vi "Multiscale Wavelet.vi"() -> ()   [LabVIEW 2023]
uses:
  SubVIs/WaveLet Param Cluster Typedef.ctl
  SubVIs/WaveLet Ramp Param Cluster Typedef.ctl
  Images/_Images.ctl
  <vilib>/addons/_Advanced Signal Processing/NI_AdvSigProcWA.lvlib
  <vilib>/vision/NI_Vision_Development_Module.lvlib
panel:
  in  "Overall Contrast":dbl=0.7
  out "Histogram Original":T1(graph)
  out "Histogram Reconstructed":T1(graph)
  in  "Multiplier":dbl[](array[slide])=[220.55384826660156, 212.6769256591797, 192.984619140625, 252.06153869628906, 283.5692443847656, 319.015380859375, 252.06153869628906, 236.3076934814453, 181.1692352294922, 110.27692413330078, 129.96923076923076, 102.4000015258789] scale=0.0..512.0
  in  "Power":dbl[](array[slide])=[0.38461539149284363, 0.4307692348957062, 0.38461539149284363, 0.5230769515037537, 0.42307692766189575, 0.5538461804389954, 0.6461538672447205, 0.6153846383094788, 0.6153846383094788, 0.6000000238418579, 0.4000000059604645, 0.4000000059604645] scale=0.0..2.0
  in  "Image":T2=enum."Part1"
  in  "Amplitudes & Widths":T3[][](array[typedef])=[[{"Amplitude"=1.0, "Width"=1.0}, {"Amplitude"=0.1, "Width"=1.0}, {"Amplitude"=0.1, "Width"=1.0}], [{"Amplitude"=1.0, "Width"=1.0}, {"Amplitude"=1.0, "Width"=1.0}, {"Amplitude"=1.0, "Width"=1.0}], [{"Amplitude"=1.0, "Width"=1.0}, {"Amplitude"=1.0, "Width"=1.0}, {"Amplitude"=1.0, "Width"=1.0}], [{"Amplitude"=1.0, "Width"=1.0}, {"Amplitude"=1.0, "Width"=1.0}, {"Amplitude"=1.0, "Width"=1.0}], [{"Amplitude"=1.0, "Width"=1.0}, {"Amplitude"=1.0, "Width"=1.0}, {"Amplitude"=1.0, "Width"=1.0}], [{"Amplitude"=1.0, "Width"=1.0}, {"Amplitude"=1.0, "Width"=1.0}, {"Amplitude"=1.0, "Width"=1.0}], [{"Amplitude"=1.0, "Width"=1.0}, {"Amplitude"=1.0, "Width"=1.0}, {"Amplitude"=1.0, "Width"=1.0}], [{"Amplitude"=1.0, "Width"=1.0}, {"Amplitude"=1.0, "Width"=1.0}, {"Amplitude"=1.0, "Width"=1.0}], [{"Amplitude"=1.0, "Width"=1.0}, {"Amplitude"=1.0, "Width"=1.0}, {"Amplitude"=1.0, "Width"=1.0}], [{"Amplitude"=1.0, "Width"=1.0}, {"Amplitude"=1.0, "Width"=1.0}, {"Amplitude"=1.0, "Width"=1.0}]]
  out "Levels":i32=9
  in  "Multipliers":T4[][](array[typedef])=[[{"Multiplier"=0.5}, {"Multiplier"=0.45}, {"Multiplier"=0.5}], [{"Multiplier"=1.0}, {"Multiplier"=1.0}, {"Multiplier"=1.0}], [{"Multiplier"=1.0}, {"Multiplier"=1.0}, {"Multiplier"=1.0}], [{"Multiplier"=1.0}, {"Multiplier"=1.0}, {"Multiplier"=1.0}], [{"Multiplier"=1.0}, {"Multiplier"=1.0}, {"Multiplier"=1.0}], [{"Multiplier"=1.0}, {"Multiplier"=1.0}, {"Multiplier"=1.0}], [{"Multiplier"=1.0}, {"Multiplier"=1.0}, {"Multiplier"=1.0}], [{"Multiplier"=1.0}, {"Multiplier"=1.0}, {"Multiplier"=1.0}], [{"Multiplier"=1.0}, {"Multiplier"=1.0}, {"Multiplier"=1.0}], [{"Multiplier"=1.0}, {"Multiplier"=1.0}, {"Multiplier"=1.0}]]
  out "Enhanced Image":T5(plugin-control)
  in  "Wavelet":u16(ring) items=["db02"=0, "db03"=1, "db04"=2, "db05"=3, "db06"=4, "db07"=5, "db08"=6, "db09"=7, "db10"=8, "db11"=9, "db12"=10, "db13"=11, "db14"=12, "Haar"=13, "bior1_3"=14, "bior1_5"=15, "bior2_2"=16, "bior2_4"=17, "bior2_6"=18, "bior2_8"=19, "bior3_1"=20, "bior3_3"=21, "bior3_5"=22, "bior3_7"=23, "bior3_9"=24, "bior4_4 (FBI)"=25, "bior5_5"=38, "bior6_8"=39, "coif1"=26, "coif2"=27, "coif3"=28, "coif4"=29, "coif5"=30, "sym2"=31, "sym3"=32, "sym4"=33, "sym5"=34, "sym6"=35, "sym7"=36, "sym8"=37]
  out "Original Image":T5(plugin-control)
  # "Multoscale Contrast Enhancement using Wavelets"
  # "HH"
  # "LH"
  # "HL"
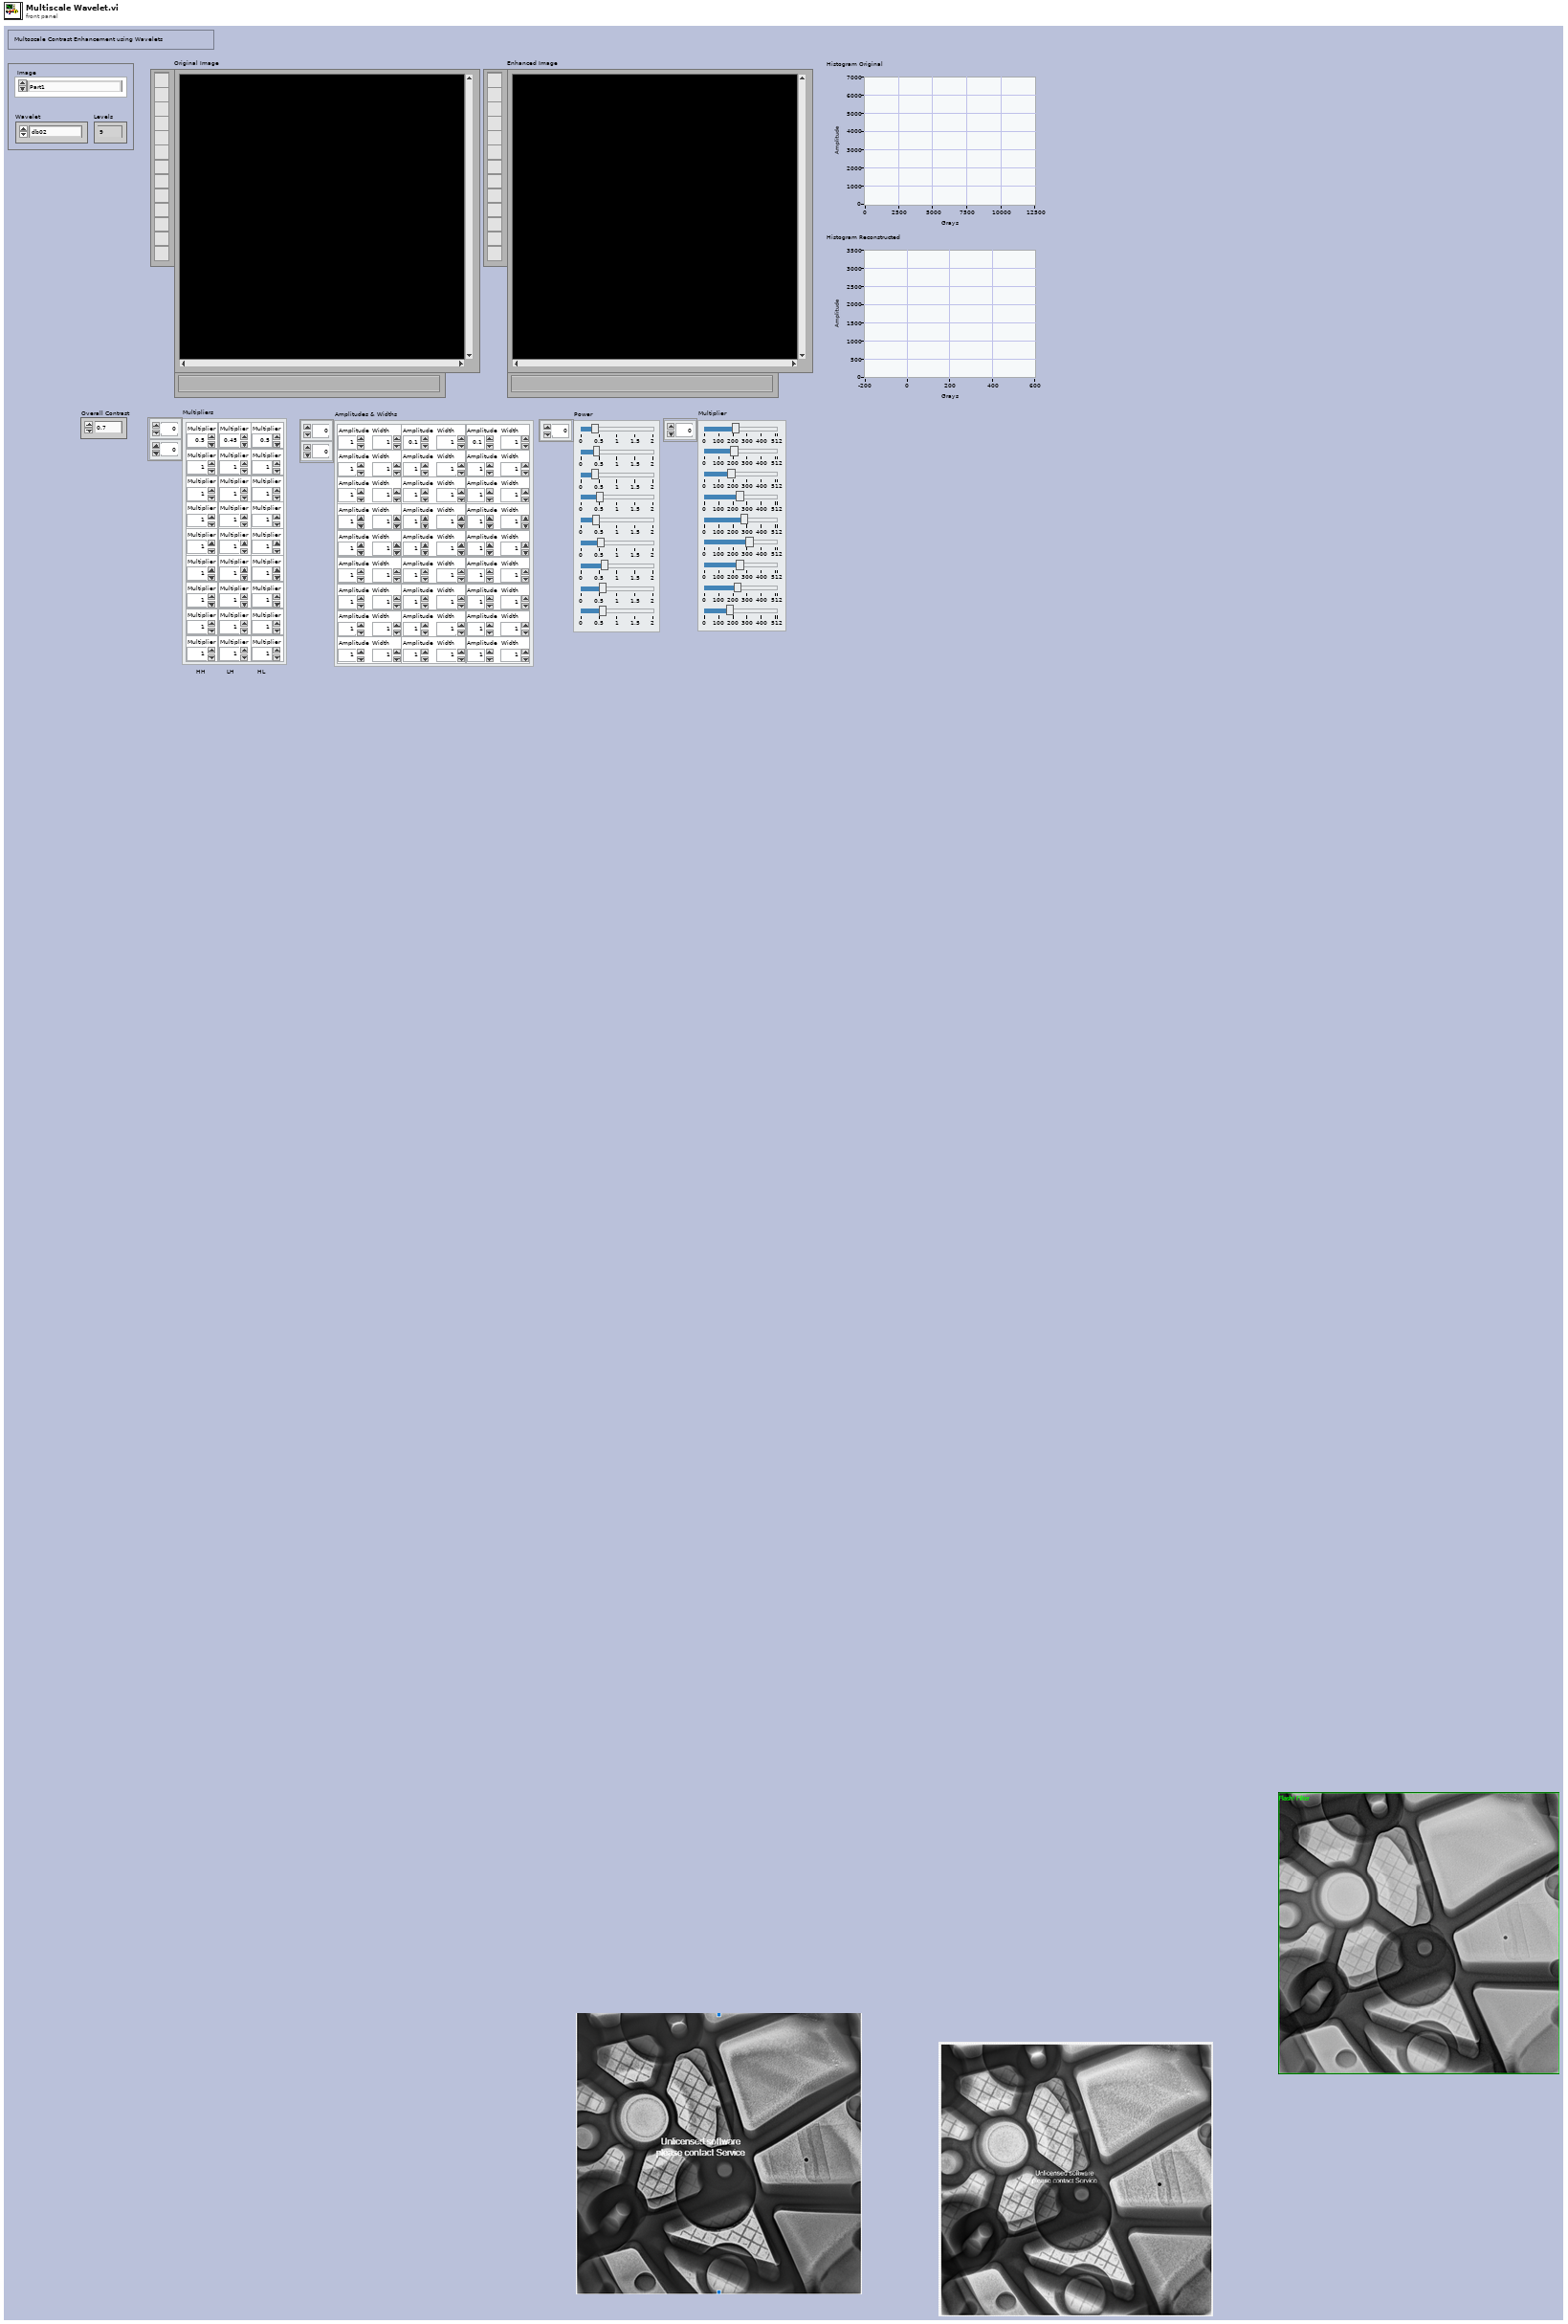
[diagram p1: front panel]
types:
  T1 = cluster{"Starting Value":sgl, "Incremental Value":sgl, "Histogram":u32[]}
  T2 = typedef "_Images.ctl" = enum16{"Balls2", "Battery1", "Battery2", "Connector1", "Subwoofer1", "Subwoofer2", "Subwoofer3", "Subwoofer4", "Hase1", "Lamp1", "Lamp2", "Mouse1", "PhotoLens1", "Po1", "PowerSupply1", "Router", "--- Step Wedges ---", "Stepwedge1", "Stepwedge2", "Stepwedge3", "--- Fusion ---", "Fusion160kV", "Fusion2-120kV", "Fusion2-320kV", "Fusion300kV", "FusionPart1-120kV", "FusionPart1-180kV", "--- PART 01 ---", "Part1", "Part2", "Part3", "Part4", "Part5", "Part6", "Part7", "Part8", "--- Different Integrations ---", "Step2737-02Int", "Step2737-04Int", "Step2737-08Int", "Step2737-16Int", "Step2737-32Int", "Step2737-64Int"}
  T3 = typedef "WaveLet Ramp Param Cluster Typedef.ctl" = cluster{"Amplitude":dbl, "Width":dbl}
  T4 = typedef "WaveLet Param Cluster Typedef.ctl" = cluster{"Multiplier":dbl}
  T5 = typedef "IMAQ Image.ctl" = refnum<image>
  T6 = typedef "Image Type" = u32
  T7 = cluster{"low_low":dbl[][], "low_high":dbl[][], "high_low":dbl[][], "high_high":dbl[][]}[]
  T8 = cluster{"low_low":dbl[][], "low_high":dbl[][], "high_low":dbl[][], "high_high":dbl[][]}
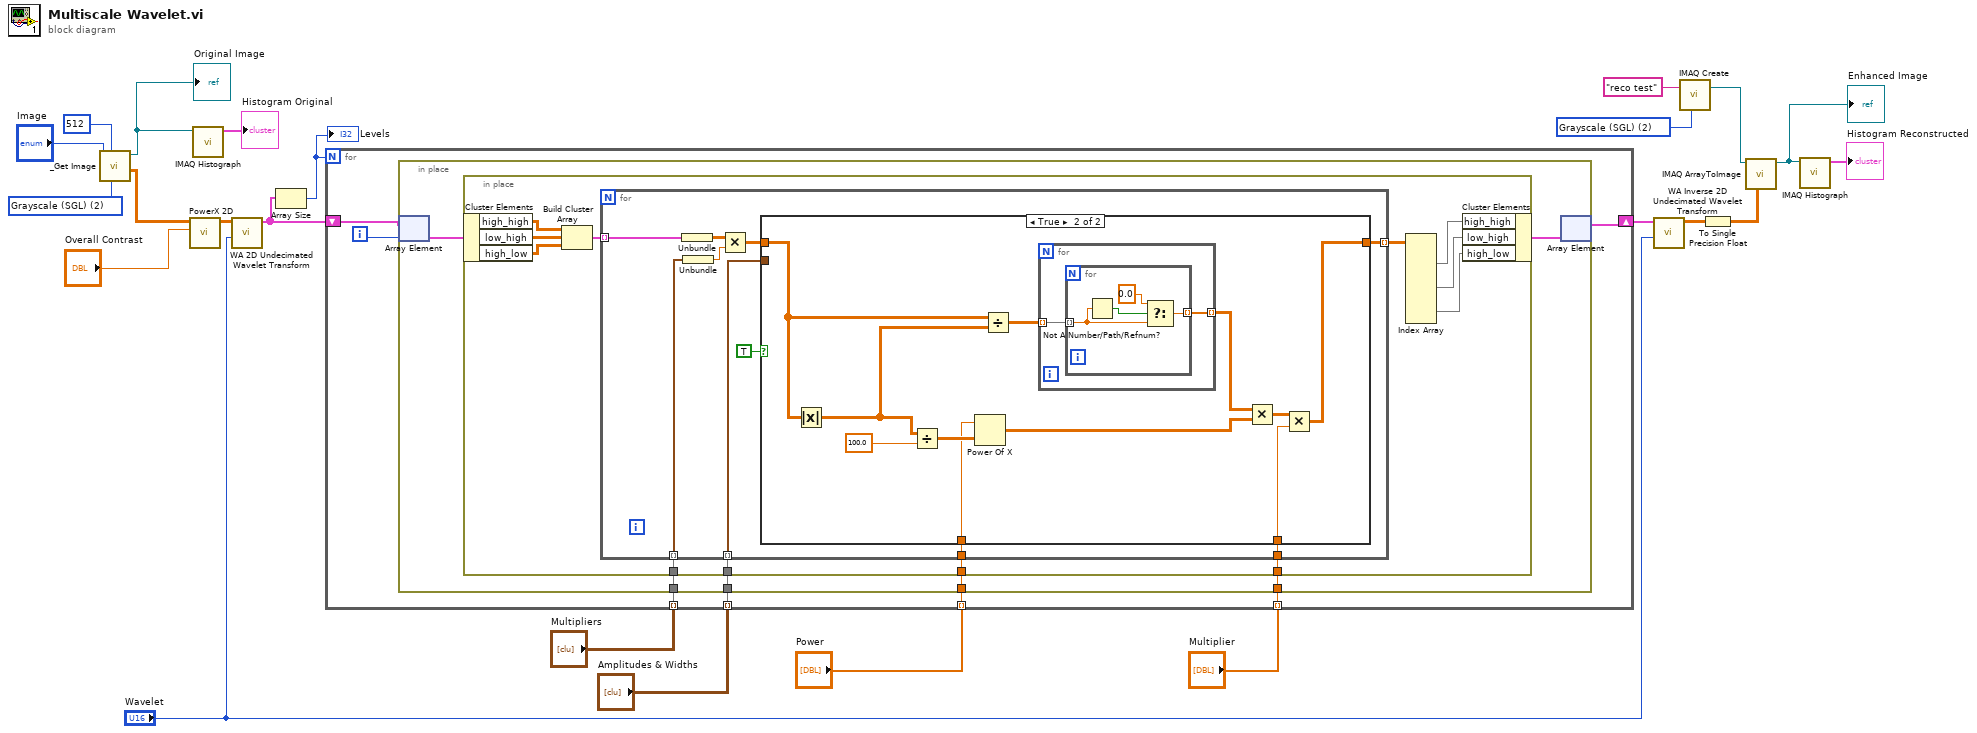
[diagram p0: block diagram]
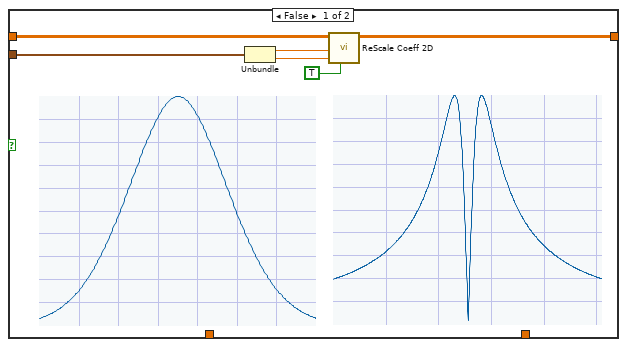
[diagram p2: hidden frame]
diagram:
  w12 = T6 2 items=["Grayscale (U8)", "Grayscale (I16)", "Grayscale (SGL)", "Complex (CSG)", "RGB (U32)", "HSL (U32)", "RGB (U64)", "Grayscale (U16)"] ("Image Type (U16)")
  w17 = T6 2 items=["Grayscale (U8)", "Grayscale (I16)", "Grayscale (SGL)", "Complex (CSG)", "RGB (U32)", "HSL (U32)", "RGB (U64)", "Grayscale (U16)"] ("Image Type")
  n1 = call "_Get Image.vi"("Image Type (U16)"=w12, "XY Resolution"=512, "Image"="Image") -> ("Image Pixels (Float)"=w4:dbl[][], "Image Out"=w2:T5)  [unwired: 5 in, 2 out]
  "Original Image" <- w2
  n2 = call "PowerX 2D.vi"("Power"="Overall Contrast", "Signal In"=w4) -> ("Signal Out"=w5:dbl[][])  [unwired: 9 in]
  n3 = call "IMAQ Histograph"("Image"=w2) -> ("Histogram Graph"=→"Histogram Original":T1)  [unwired: 7 in, 3 out]
  n4 = call <vilib>:"WA 2D Undecimated Wavelet Transform.vi"("wavelet"="Wavelet", "signal"=w5) -> ("UWT coef"=w14:T7)  [unwired: 3 in, 6 out]
  n5 = Array Size(array=w14) -> (size(s)=w20:i32)
  "Levels" <- w20
  n6 = for {
    N: w20 -> [_]
    shift-right: [w24] -> w16
    shift-left: w14 -> [w26]
    tunnel: "Multipliers" -> [w30] mode=indexing
    tunnel: "Amplitudes & Widths" -> [w29] mode=indexing
    tunnel: "Power" -> [w28] mode=indexing
    tunnel: "Multiplier" -> [w27] mode=indexing
    i -> [w25]
    n7 = in-place {
      in-place-border: w30 -> [w36]
      in-place-border: w29 -> [w35]
      in-place-border: w28 -> [w34]
      in-place-border: w27 -> [w33]
      n8 = in-place-array #1(w26, w25) -> (w32:T8)
      n9 = in-place {
        in-place-border: w36 -> [w46]
        in-place-border: w35 -> [w45]
        in-place-border: w34 -> [w44]
        in-place-border: w33 -> [w43]
        n10 = in-place-cluster #2(w32) -> ("high_high"=w42:dbl[][], "low_high"=w41:dbl[][], "high_low"=w40:dbl[][])
        n11 = Build Cluster Array(w42, w41, w40) -> (w48:cluster{"high_low":dbl[][]}[])
        n12 = for {
          tunnel: w48 -> [w58] mode=indexing
          tunnel: [w53] -> w47 mode=indexing
          tunnel: w46 -> [w55] mode=indexing
          tunnel: w45 -> [w56] mode=indexing
          tunnel: w44 -> [w52]
          tunnel: w43 -> [w51]
          n13 = Unbundle(w58) -> ("high_low"=w57:dbl[][])
          n14 = Unbundle(w55) -> ("Multiplier"=w50:dbl)
          n15 = Multiply(x=w57, y=w50) -> (x*y=w54:dbl[][])
          n16 = case shown="True" TRUE {
            tunnel: w56 -> [w59 _]
            tunnel: w54 -> [w61 w69]
            tunnel: [w60 w68] -> w53
            tunnel: w52 -> [_ w67]
            tunnel: w51 -> [_ w66]
            frame False {
              n17 = Unbundle(w59) -> ("Amplitude"=w64:dbl, "Width"=w63:dbl)
              n18 = call "ReScale Coeff 2D.vi"("Gauss"=TRUE, "amplitude"=w64, "Width"=w63, "Array in"=w61) -> ("Array out"=w60:dbl[][])  [unwired: 7 in]
            }
            frame True {
              n19 = Absolute Value(x=w69) -> (abs(x)=w75:dbl[][])
              n20 = Divide(x=w75, y=sgl 100.0) -> (x/y=w71:dbl[][])
              n21 = Power Of X(1:w71, 2:w67) -> (0:w70:dbl[][])
              n22 = Divide(x=w69, y=w75) -> (x/y=w73:dbl[][])
              n23 = for {
                tunnel: w73 -> [w77] mode=indexing
                tunnel: [w76] -> w72 mode=indexing
                n24 = for {
                  tunnel: w77 -> [w79] mode=indexing
                  tunnel: [w80] -> w76 mode=indexing
                  n25 = Not A Number/Path/Refnum?(number/path/refnum=w79) -> (NaN/Path/Refnum?=w78:bool)
                  n26 = Select(t=0.0, s=w78, f=w79) -> (s? t:f=w80:dbl)
                }
              }
              n27 = Multiply(x=w72, y=w70) -> (x*y=w74:dbl[][])
              n28 = Multiply(x=w74, y=w66) -> (x*y=w68:dbl[][])
            }
          }
        }
        n29 = Index Array(array=w47) -> (element #1=w39:dbl[][], element #2=w38:dbl[][], element #3=w37:dbl[][])  [unwired: 9 in]
        n30 = in-place-cluster #2("high_high"=w39, "low_high"=w38, "high_low"=w37) -> (w31:T8)
      }
      n31 = in-place-array #1(w31) -> (w24:T7)  [unwired: 1 out]
    }
  }
  n32 = call <vilib>:"WA Inverse 2D Undecimated Wavelet Transform.vi"("wavelet"="Wavelet", "UWT coef"=w16) -> ("signal"=w19:dbl[][])  [unwired: 2 in, 7 out]
  n33 = call "IMAQ Create"("Image Name"="reco test", "Image Type"=w17) -> ("New Image"=w23:T5)  [unwired: 3 in, 1 out]
  n34 = To Single Precision Float(number=w19) -> (single precision float=w3:sgl[][])
  n35 = call "IMAQ ArrayToImage"("Image Pixels (Float)"=w3, "Image"=w23) -> ("Image Out"=w1:T5)  [unwired: 8 in, 1 out]
  "Enhanced Image" <- w1
  n36 = call "IMAQ Histograph"("Image"=w1) -> ("Histogram Graph"=→"Histogram Reconstructed":T1)  [unwired: 7 in, 3 out]
